vi "ReadUnbundler.vi"(1 "reference":refnum<vi>) -> (0 "Unbundler":T6)   [LabVIEW 2013]
uses:
  <vilib>/Utility/miscctls.llb/LVBoundsTypeDef.ctl
  <vilib>/Utility/miscctls.llb/LVPositionTypeDef.ctl
  <vilib>/Utility/miscctls.llb/LVRectTypeDef.ctl
  <vilib>/Utility/miscctls.llb/LVBreakpointStatusEnum.ctl
  <vilib>/picture/picture.llb/imagedata.ctl
panel:
  out "error out 23":errorcluster
  out "error out 22":errorcluster
  out "error out 21":errorcluster
  out "error out 20":errorcluster
  out "error out 19":errorcluster
  out "error out 18":errorcluster
  out "error out 17":errorcluster
  out "error out 16":errorcluster
  out "error out 15":errorcluster
  out "error out 14":errorcluster
  out "error out 13":errorcluster
  out "error out 12":errorcluster
  out "error out 11":errorcluster
  out "error out 10":errorcluster
  out "error out 9":errorcluster
  out "error out 8":errorcluster
  out "error out 7":errorcluster
  out "error out 6":errorcluster
  out "error out 5":errorcluster
  out "error out 4":errorcluster
  out "error out 3":errorcluster
  out "error out 2":errorcluster
  out "error out":errorcluster
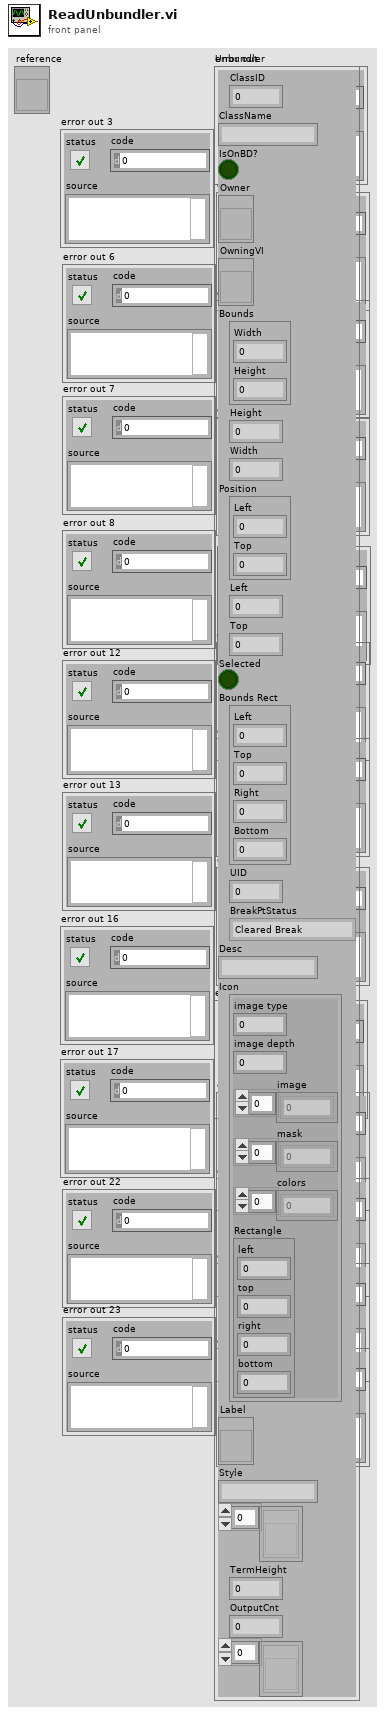
[diagram p1: front panel]
types:
  T1 = typedef "LVBoundsTypeDef.ctl" = cluster{"Width":u32, "Height":u32}
  T2 = typedef "LVPositionTypeDef.ctl" = cluster{"Left":i32, "Top":i32}
  T3 = typedef "LVRectTypeDef.ctl" = cluster{"Left":i16, "Top":i16, "Right":i16, "Bottom":i16}
  T4 = typedef "LVBreakpointStatusEnum.ctl" = enum8{"Cleared Break", "Enabled Break", "Disabled Break"}
  T5 = typedef "imagedata.ctl" = cluster{"image type":i32, "image depth":i32, "image":u8[], "mask":u8[], "colors":u32[], "Rectangle":cluster{"left":i16, "top":i16, "right":i16, "bottom":i16}}
  T6 = cluster{"ClassID":u32, "ClassName":string, "IsOnBD?":bool, "Owner":refnum<vi>, "OwningVI":refnum<vi>, "Bounds":T1, "Height":u32, "Width":u32, "Position":T2, "Left":i32, "Top":i32, "Selected":bool, "Bounds Rect":T3, "UID":i32, "BreakPtStatus":T4, "Desc":string, "Icon":T5, "Label":refnum<vi>, "Style":string, "Terms[]":refnum<vi>[], "TermHeight":i32, "OutputCnt":i32, "OutputTerms[]":refnum<vi>[]}
  T7 = cluster{"ClassID":u32, "ClassName":string, "IsOnBD?":bool, "Owner":refnum<vi>, "OwningVI":refnum<vi>, "Bounds":T1, "Height":u32, "Width":u32, "Position":T2, "Left":i32, "Top":i32, "Selected":bool, "Bounds Rect":T3, "UID":i32, "BreakPtStatus":T4, "Desc":string, "Icon":T5, "Label":refnum<vi>, "Style":string, refnum<vi>[], "TermHeight":i32, "OutputCnt":i32, refnum<vi>[]}
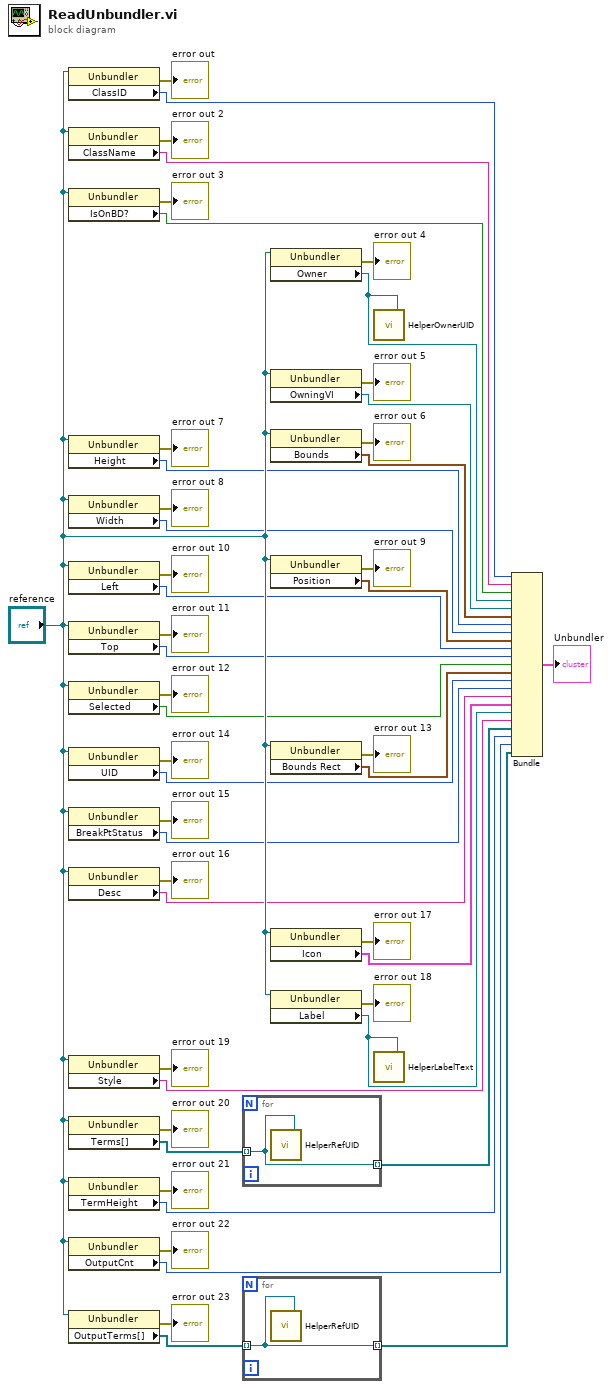
[diagram p0: block diagram]
diagram:
  n1 = property class="Unbundler"(reference="reference") -> (error out=→"error out":errorcluster, "ClassID"=w48:u32)  [unwired: 1 in, 1 out]
  n2 = property class="Unbundler"(reference="reference") -> (error out=→"error out 2":errorcluster, "ClassName"=w46:string)  [unwired: 1 in, 1 out]
  n3 = property class="Unbundler"(reference="reference") -> (error out=→"error out 3":errorcluster, "IsOnBD?"=w44:bool)  [unwired: 1 in, 1 out]
  n4 = property class="Unbundler"(reference="reference") -> (error out=→"error out 7":errorcluster, "Height"=w36:u32)  [unwired: 1 in, 1 out]
  n5 = property class="Unbundler"(reference="reference") -> (error out=→"error out 8":errorcluster, "Width"=w34:u32)  [unwired: 1 in, 1 out]
  n6 = property class="Unbundler"(reference="reference") -> (error out=→"error out 10":errorcluster, "Left"=w30:i32)  [unwired: 1 in, 1 out]
  n7 = property class="Unbundler"(reference="reference") -> (error out=→"error out 11":errorcluster, "Top"=w28:i32)  [unwired: 1 in, 1 out]
  n8 = property class="Unbundler"(reference="reference") -> (error out=→"error out 12":errorcluster, "Selected"=w26:bool)  [unwired: 1 in, 1 out]
  n9 = property class="Unbundler"(reference="reference") -> (error out=→"error out 14":errorcluster, "UID"=w22:i32)  [unwired: 1 in, 1 out]
  n10 = property class="Unbundler"(reference="reference") -> (error out=→"error out 15":errorcluster, "BreakPtStatus"=w20:T4)  [unwired: 1 in, 1 out]
  n11 = property class="Unbundler"(reference="reference") -> (error out=→"error out 16":errorcluster, "Desc"=w18:string)  [unwired: 1 in, 1 out]
  n12 = property class="Unbundler"(reference="reference") -> (error out=→"error out 19":errorcluster, "Style"=w12:string)  [unwired: 1 in, 1 out]
  n13 = property class="Unbundler"(reference="reference") -> (error out=→"error out 20":errorcluster, "Terms[]"=w10:refnum<vi>[])  [unwired: 1 in, 1 out]
  n14 = property class="Unbundler"(reference="reference") -> (error out=→"error out 21":errorcluster, "TermHeight"=w7:i32)  [unwired: 1 in, 1 out]
  n15 = property class="Unbundler"(reference="reference") -> (error out=→"error out 22":errorcluster, "OutputCnt"=w5:i32)  [unwired: 1 in, 1 out]
  n16 = property class="Unbundler"(reference="reference") -> (error out=→"error out 23":errorcluster, "OutputTerms[]"=w3:refnum<vi>[])  [unwired: 1 in, 1 out]
  n17 = for {
    tunnel: w10 -> [w51] mode=indexing
    tunnel: [w51] -> w9 mode=indexing
    n18 = call "HelperRefUID.vi"("Text in"=w51) -> ()  [unwired: 1 out]
  }
  n19 = for {
    tunnel: w3 -> [w52] mode=indexing
    tunnel: [w52] -> w2 mode=indexing
    n20 = call "HelperRefUID.vi"("Text in"=w52) -> ()  [unwired: 1 out]
  }
  n21 = property class="Unbundler"(reference="reference") -> (error out=→"error out 4":errorcluster, "Owner"=w42:refnum<vi>)  [unwired: 1 in, 1 out]
  n22 = property class="Unbundler"(reference="reference") -> (error out=→"error out 5":errorcluster, "OwningVI"=w40:refnum<vi>)  [unwired: 1 in, 1 out]
  n23 = property class="Unbundler"(reference="reference") -> (error out=→"error out 6":errorcluster, "Bounds"=w38:T1)  [unwired: 1 in, 1 out]
  n24 = property class="Unbundler"(reference="reference") -> (error out=→"error out 9":errorcluster, "Position"=w32:T2)  [unwired: 1 in, 1 out]
  n25 = property class="Unbundler"(reference="reference") -> (error out=→"error out 13":errorcluster, "Bounds Rect"=w24:T3)  [unwired: 1 in, 1 out]
  n26 = property class="Unbundler"(reference="reference") -> (error out=→"error out 17":errorcluster, "Icon"=w16:T5)  [unwired: 1 in, 1 out]
  n27 = property class="Unbundler"(reference="reference") -> (error out=→"error out 18":errorcluster, "Label"=w14:refnum<vi>)  [unwired: 1 in, 1 out]
  n28 = call "HelperOwnerUID.vi"("Generic in"=w42) -> ()  [unwired: 1 out]
  n29 = call "HelperLabelText.vi"("Text in"=w14) -> ()  [unwired: 1 out]
  n30 = Bundle("ClassID"=w48, "ClassName"=w46, "IsOnBD?"=w44, "Owner"=w42, "OwningVI"=w40, "Bounds"=w38, "Height"=w36, "Width"=w34, "Position"=w32, "Left"=w30, "Top"=w28, "Selected"=w26, "Bounds Rect"=w24, "UID"=w22, "BreakPtStatus"=w20, "Desc"=w18, "Icon"=w16, "Label"=w14, "Style"=w12, w9, "TermHeight"=w7, "OutputCnt"=w5, w2) -> (→"Unbundler":T7)  [unwired: 1 in]
